vi "PurePursuitPathSearch.vi"(4 "Look-Ahead Time (s)":dbl=0.25, 6 "Search Window (s)":dbl=2.0, 8 "Robot Y (in)":dbl, 9 "Robot X (in)":dbl, 10 "Reint":bool, 11 "Path":dbl[][](array[numeric])) -> (0 "Angle Goal (deg)":dbl, 1 "Velocity Goal (in/s)":dbl, 2 "Angle To Goal (deg)":dbl, 3 "Distance to Goal (in)":dbl, 5 "Distance from End (in)":dbl, 7 "Distance from Start (in)":dbl)   [LabVIEW 2019]
doc: "Finds the point on the path closest to the robot's current position. This VI is designed to integrate with a pure pursuit path following algorithm. It outputs the robot's distance and angle to the pursuit point, along with the target velocity, goal orientation, and the distances from the path end points."
panel:
  out "Look-Ahead Point":i32
  out "Closest Point":i32
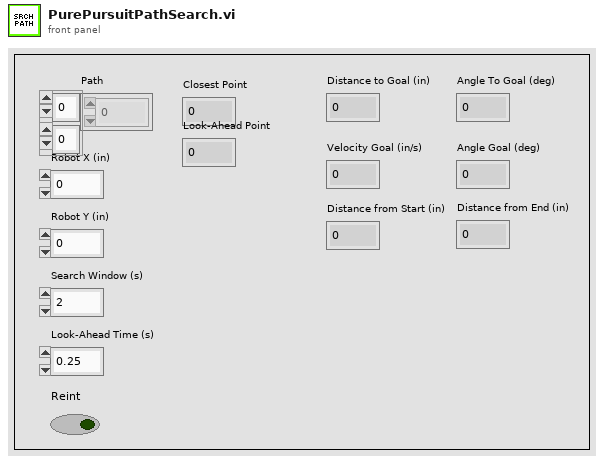
[diagram p1: front panel]
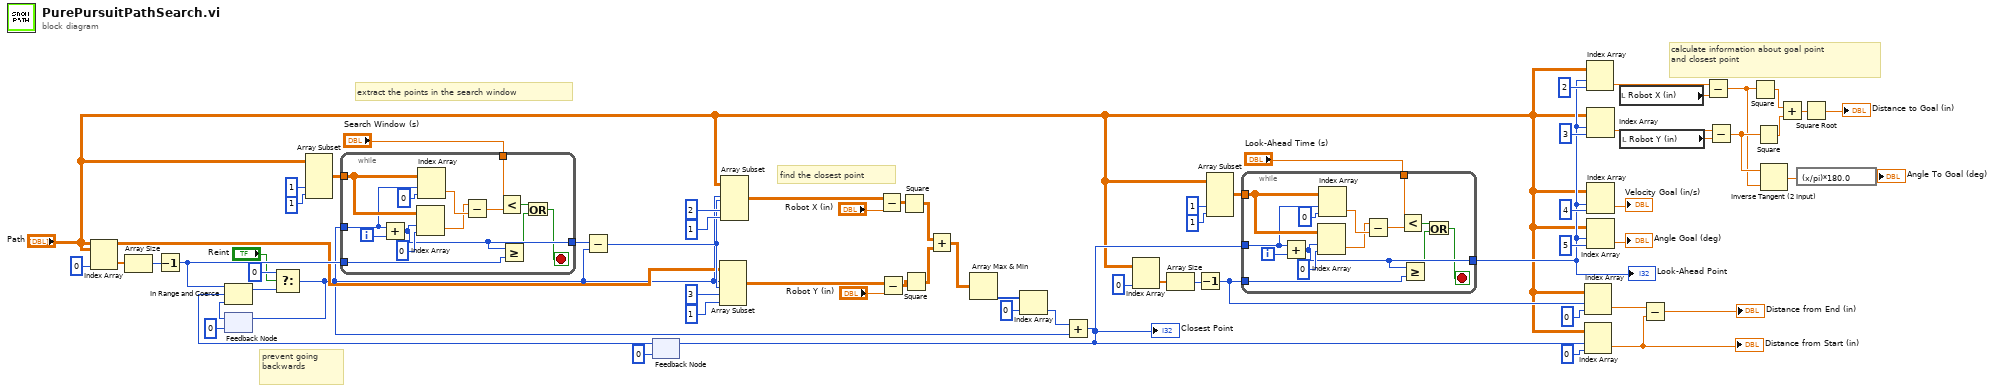
[diagram p0: block diagram]
diagram:
  # "calculate information about goal point\nand closest point"
  # "prevent going \nbackwards"
  # "find the closest point"
  # "extract the points in the search window"
  n1 = Index Array(array="Path", index (col)=0 ("disabled index (col)")) -> (element=w30:dbl[])  [unwired: 1 in]
  n2 = Array Size(array=w30) -> (size(s)=w31:i32)
  n3 = Decrement(x=w31) -> (x-1=w27:i32)
  n4 = feedback #1(0) -> (w28:i32)
  n5 = Array Subset(array="Path", index (col)=1 ("index"), length (col)=1 ("length")) -> (w51:dbl[][])  [unwired: 2 in]
  n6 = feedback #2(0) -> (w26:i32)
  n7 = In Range and Coerce(upper limit=w27, x=w26, lower limit=w28) -> (coerced(x)=w4:i32)  [unwired: 1 out]
  n8 = Select(t=0, s="Reint", f=w4) -> (s? t:f=w3:i32)
  n9 = feedback-in #1(w3) -> ()
  n10 = while {
    tunnel: w3 -> [w79]
    tunnel: w51 -> [w80]
    tunnel: "Search Window (s)" -> [w74]
    tunnel: [w73] -> w49
    tunnel: w27 -> [w69]
    i -> [w82]
    stop <- w71 stop-if-true
    # "Search window"
    n11 = Add(x=w79, y=w82) -> (x+y=w73:i32)
    n12 = Index Array(array=w80, index (row)=w73, index (col)=0 ("disabled index (col)")) -> (element=w76:dbl)
    n13 = Index Array(array=w80, index (row)=w79, index (col)=0 ("disabled index (col)")) -> (element=w77:dbl)
    n14 = Subtract(x=w76, y=w77) -> (x-y=w75:dbl)
    n15 = Less?(x=w74, y=w75) -> (x < y?=w72:bool)
    n16 = Greater Or Equal?(x=w73, y=w69) -> (x >= y?=w70:bool)
    n17 = Or(x=w72, y=w70) -> (x .or. y?=w71:bool)
  }
  n18 = Subtract(x=w49, y=w3) -> (x-y=w48:i32)
  n19 = Array Subset(array="Path", index (row)=w3, length (row)=w48, index (col)=3 ("index"), length (col)=1 ("length")) -> (w60:dbl[][])
  n20 = Array Subset(array="Path", index (row)=w3, length (row)=w48, index (col)=2 ("index"), length (col)=1 ("length")) -> (w66:dbl[][])
  n21 = Subtract(x=w66, y="Robot X (in)") -> (x-y=w65:dbl[][])
  n22 = Subtract(x=w60, y="Robot Y (in)") -> (x-y=w61:dbl[][])
  n23 = Square(x=w65) -> (x^2=w58:dbl[][])
  n24 = Square(x=w61) -> (x^2=w57:dbl[][])
  n25 = Add(x=w58, y=w57) -> (x+y=w56:dbl[][])
  n26 = Array Max & Min(array=w56) -> (min index (indices)=w55:i32[])  [unwired: 3 out]
  n27 = Index Array(array=w55, index=0) -> (element=w47:i32)
  n28 = Add(x=w47, y=w3) -> (x+y=w13:i32)
  "Closest Point" <- w13
  n29 = feedback-in #2(w13) -> ()
  n30 = Index Array(array="Path", index (col)=0 ("disabled index (col)")) -> (element=w20:dbl[])  [unwired: 1 in]
  n31 = Array Size(array=w20) -> (size(s)=w12:i32)
  n32 = Decrement(x=w12) -> (x-1=w10:i32)
  n33 = Array Subset(array="Path", index (col)=1 ("index"), length (col)=1 ("length")) -> (w22:dbl[][])  [unwired: 2 in]
  n34 = while {
    tunnel: w13 -> [w93]
    tunnel: w22 -> [w94]
    tunnel: "Look-Ahead Time (s)" -> [w88]
    tunnel: [w87] -> w14
    tunnel: w10 -> [w83]
    i -> [w96]
    stop <- w85 stop-if-true
    # "Search window"
    n35 = Add(x=w93, y=w96) -> (x+y=w87:i32)
    n36 = Index Array(array=w94, index (row)=w87, index (col)=0 ("disabled index (col)")) -> (element=w90:dbl)
    n37 = Index Array(array=w94, index (row)=w93, index (col)=0 ("disabled index (col)")) -> (element=w91:dbl)
    n38 = Subtract(x=w90, y=w91) -> (x-y=w89:dbl)
    n39 = Less?(x=w88, y=w89) -> (x < y?=w86:bool)
    n40 = Greater Or Equal?(x=w87, y=w83) -> (x >= y?=w84:bool)
    n41 = Or(x=w86, y=w84) -> (x .or. y?=w85:bool)
  }
  "Look-Ahead Point" <- w14
  n42 = Index Array(array="Path", index (row)=w10, index (col)=0 ("disabled index (row)")) -> (element=w8:dbl)
  n43 = Index Array(array="Path", index (row)=w13, index (col)=0 ("disabled index (col)")) -> (element=w6:dbl)
  "Distance from Start (in)" <- w6
  n44 = Index Array(array="Path", index (row)=w14, index (col)=2 ("disabled index (col)")) -> (element=w44:dbl)
  n45 = Index Array(array="Path", index (row)=w14, index (col)=3 ("disabled index (col)")) -> (element=w42:dbl)
  n46 = Index Array(array="Path", index (row)=w14, index (col)=4 ("disabled index (col)")) -> (element=→"Velocity Goal (in/s)":dbl)
  n47 = Index Array(array="Path", index (row)=w14, index (col)=5 ("disabled index (col)")) -> (element=→"Angle Goal (deg)":dbl)
  n48 = local read "Robot X (in)"() -> (w43:dbl)
  n49 = local read "Robot Y (in)"() -> (w41:dbl)
  n50 = Subtract(x=w8, y=w6) -> (x-y=→"Distance from End (in)":dbl)
  n51 = Subtract(x=w44, y=w43) -> (x-y=w35:dbl)
  n52 = Subtract(x=w42, y=w41) -> (x-y=w36:dbl)
  n53 = Square(x=w35) -> (x^2=w39:dbl)
  n54 = Square(x=w36) -> (x^2=w40:dbl)
  n55 = Inverse Tangent (2 Input)(1:w35, 2:w36) -> (0:w34:dbl)
  n56 = Add(x=w39, y=w40) -> (x+y=w38:dbl)
  n57 = expression code="(x/pi)*180.0"(w34) -> (→"Angle To Goal (deg)":dbl)
  n58 = Square Root(x=w38) -> (sqrt(x)=→"Distance to Goal (in)":dbl)
